vi "产品界面.vi"(8 "错误输入（无错误）":errorcluster, 10 "界面切换队列":refnum<queue>, 11 "VISA资源名称输入":refnum<visa-resource-name>) -> (0 "错误输出":errorcluster, 3 "VISA资源名称输出":refnum<visa-resource-name>)   [LabVIEW 2018]
panel:
  out "毫秒计时值":u32
  in  "枚举":T1(ring)
  in  "选项卡控件":enum32{"选项卡 1", "选项卡 2"}(tab)
  out "写DT200+主料盘参数界面":bool
  out "写DT203":bool
  out "写R176+读R177":bool
  in  "DT422":u16(ring) items=["禁用值", "无名称1", "无名称2", "无名称3", "无名称4", "无名称5", "无名称6", "无名称7", "无名称8", "无名称9", "无名称10", "无名称11", "无名称12", "无名称13", "无名称14", "无名称15", "无名称16", "无名称17", "无名称18", "无名称19", "无名称20", "无名称21", "无名称22", "无名称23", "无名称24", "无名称25", "无名称26", "无名称27", "无名称28", "无名称29", "无名称30", "无名称31", "无名称32", "无名称33", "无名称34", "无名称35", "无名称36", "无名称37", "无名称38", "无名称39", "无名称40", "无名称41", "无名称42", "无名称43", "无名称44", "无名称45", "无名称46", "无名称47", "无名称48", "无名称49", "无名称50", "无名称51", "无名称52", "无名称53", "无名称54", "无名称55", "无名称56", "无名称57", "无名称58", "无名称59", "55UYFJJI"]
  in  "DT420":u16(ring) items=["禁用值", "无名称1", "无名称2", "无名称3", "无名称4", "无名称5", "无名称6", "无名称7", "无名称8", "无名称9", "无名称10", "无名称11", "无名称12", "无名称13", "无名称14", "无名称15", "无名称16", "无名称17", "无名称18", "无名称19", "无名称20", "无名称21", "无名称22", "无名称23", "无名称24", "无名称25", "无名称26", "无名称27", "无名称28", "无名称29", "无名称30", "无名称31", "无名称32", "无名称33", "无名称34", "无名称35", "无名称36", "无名称37", "无名称38", "无名称39", "无名称40", "无名称41", "无名称42", "无名称43", "无名称44", "无名称45", "无名称46", "无名称47", "无名称48", "无名称49", "无名称50", "无名称51", "无名称52", "无名称53", "无名称54", "无名称55", "无名称56", "无名称57", "无名称58", "无名称59", "55UYFJJI"]
  out "字符串 2":string
  in  "产品名称":u16(ring) items=["禁用值", "无名称1", "无名称2", "无名称3", "无名称4", "无名称5", "无名称6", "无名称7", "无名称8", "无名称9", "无名称10", "无名称11", "无名称12", "无名称13", "无名称14", "无名称15", "无名称16", "无名称17", "无名称18", "无名称19", "无名称20", "无名称21", "无名称22", "无名称23", "无名称24", "无名称25", "无名称26", "无名称27", "无名称28", "无名称29", "无名称30", "无名称31", "无名称32", "无名称33", "无名称34", "无名称35", "无名称36", "无名称37", "无名称38", "无名称39", "无名称40", "无名称41", "无名称42", "无名称43", "无名称44", "无名称45", "无名称46", "无名称47", "无名称48", "无名称49", "无名称50", "无名称51", "无名称52", "无名称53", "无名称54", "无名称55", "无名称56", "无名称57", "无名称58", "无名称59", "55UYFJJI"]
  out "DDT90356":dbl
  out "DDT90348":dbl
  out "自动界面":bool
  out "手动界面":bool
  out "参数界面":bool
  out "IO界面":bool
  out "产品界面":bool
  out "字符串":string
  out "DDT90352":dbl
  out "DDT90360":dbl
  out "DT1184":T2(ring)
  out "通讯周期":dbl
  out "数值":dbl
  # "X"
  # "Z1"
  # "XXXXX自动化设备有限公司"
  # "Z2"
  # "Y"
  # "调用"
  # "设置"
  # "编号"
  # "名称"
  # "将产品"
  # "复制到"
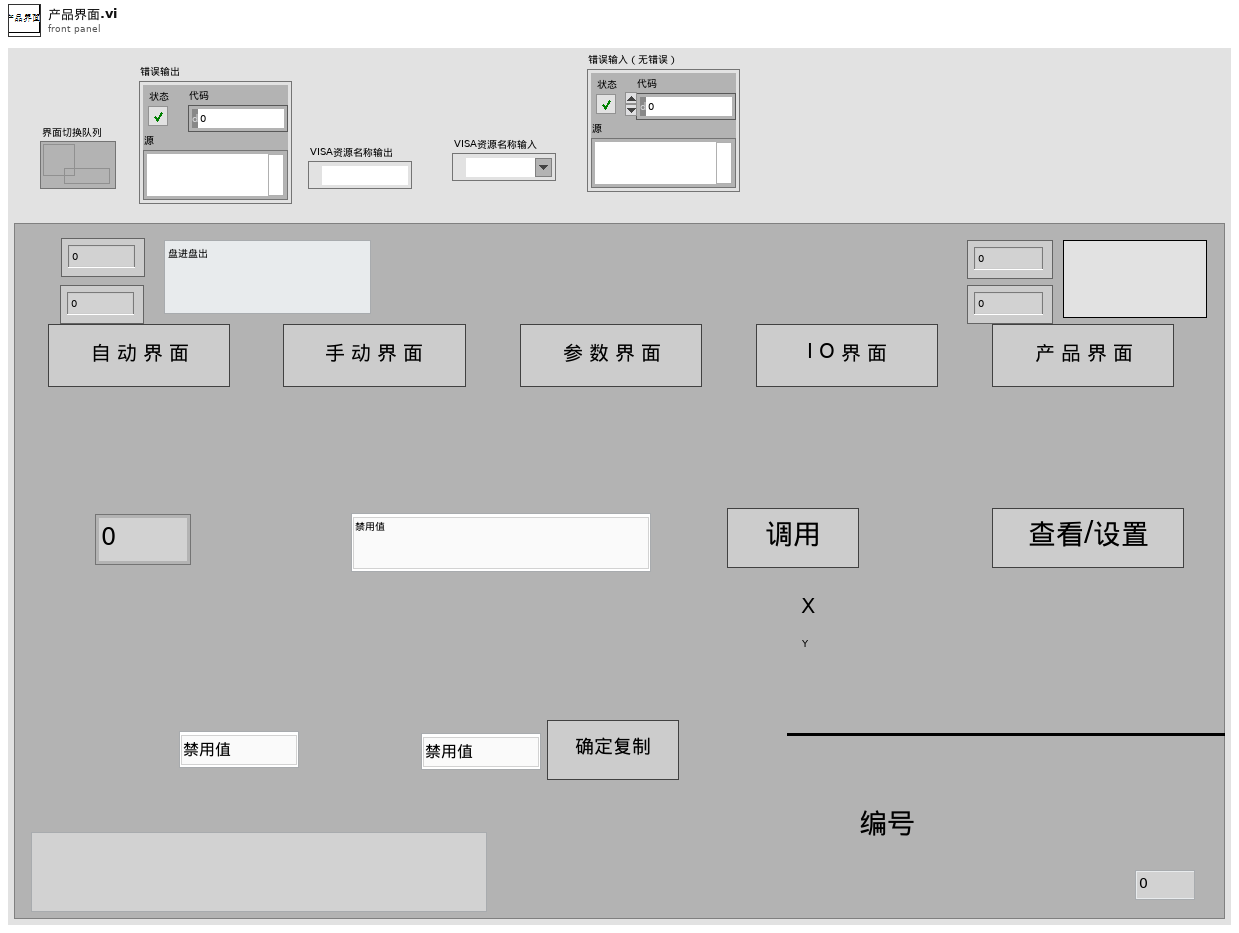
[diagram p1: front panel]
types:
  T1 = enum16{"读初始化", "读R166+8", "读DT420+10", "读R177+8", "读DDT90356", "读DT1184", "读DDT90348", ""}
  T2 = enum16{"盘进盘出", "卷进卷出", "盘进卷出", "管进盘出", "管进卷出", "卷进盘出", ""}
  T3 = enum8{"Enabled", "Disabled", "Disabled and Grayed Out"}
  T4 = typedef "数据簇.ctl" = cluster{"字符串":string, "数值":i32, "布尔":bool}
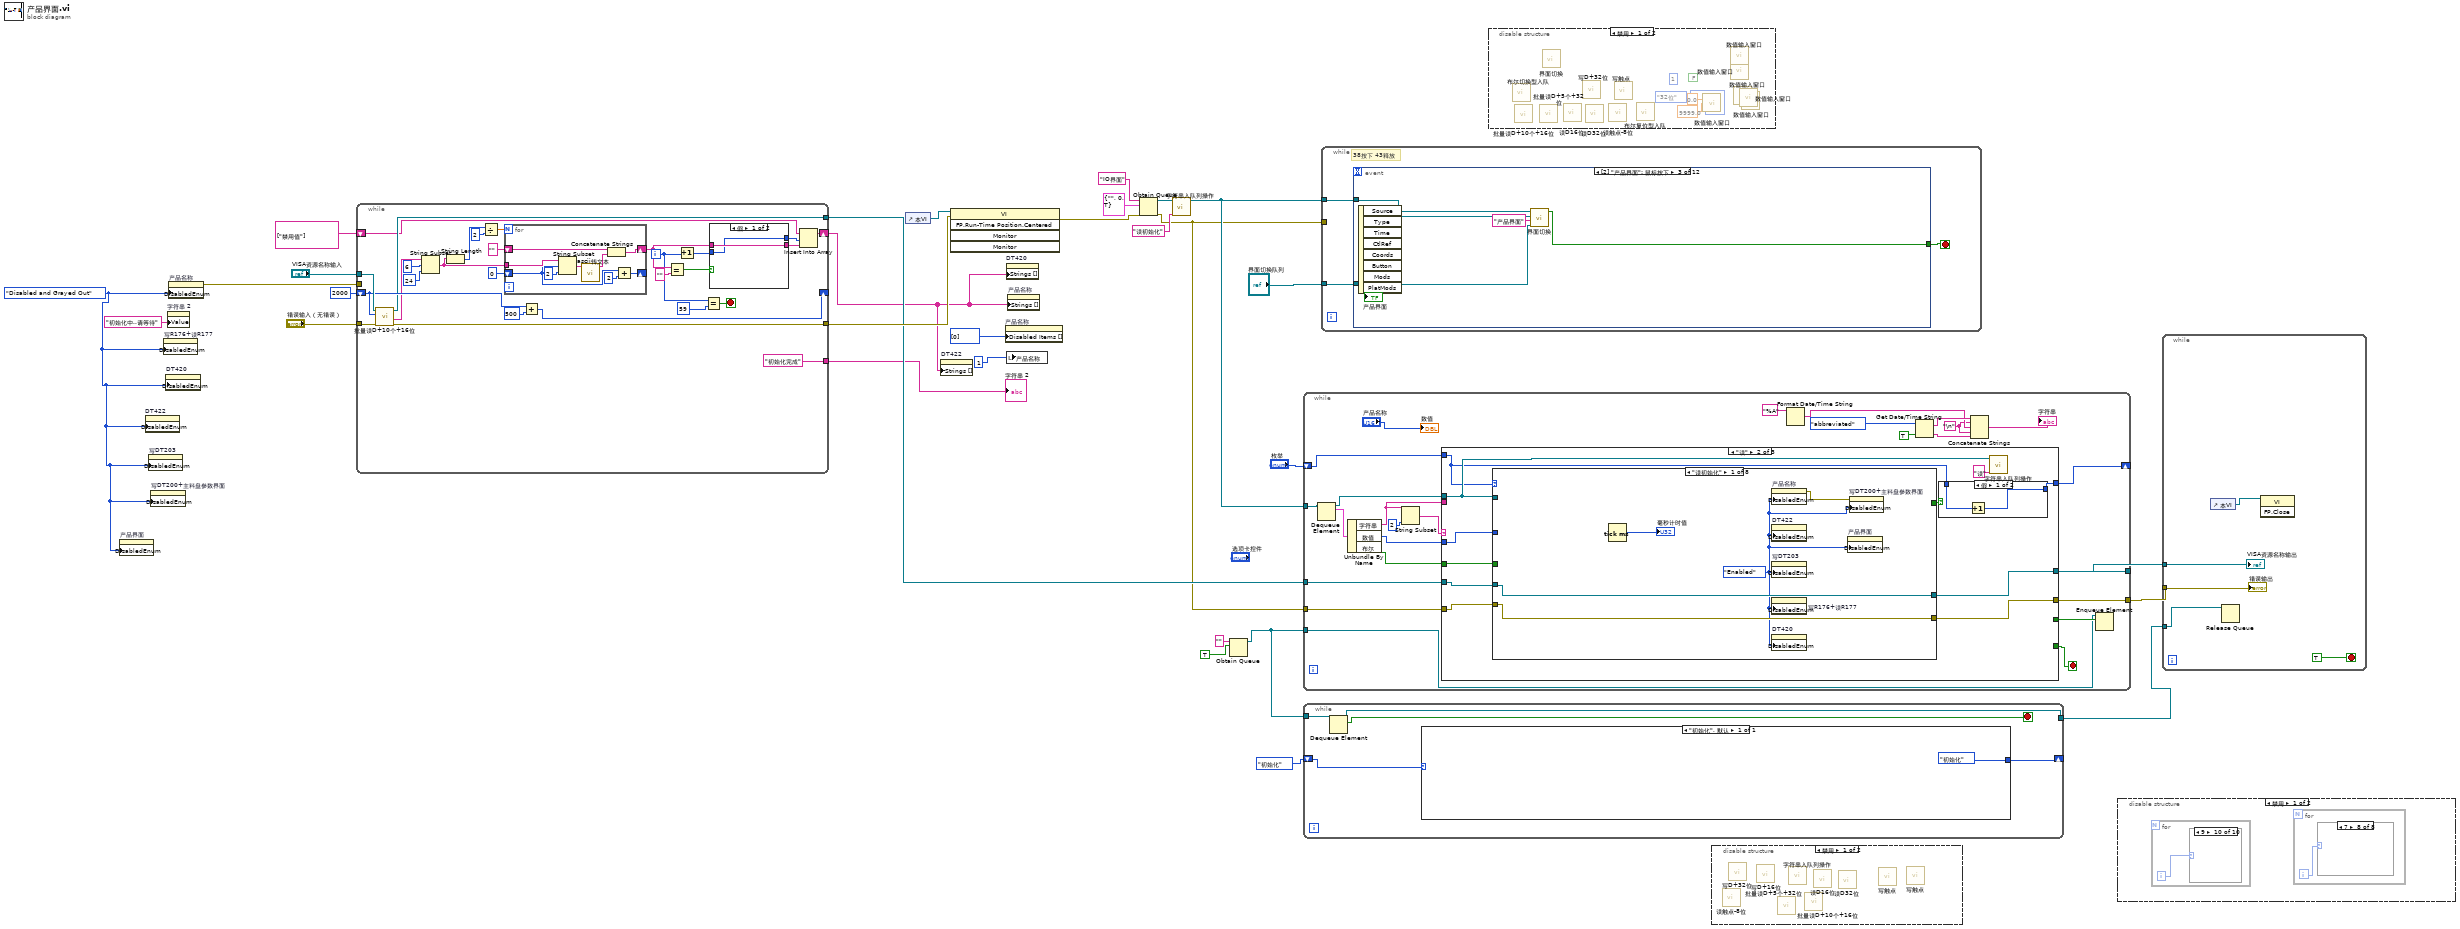
[diagram p0: block diagram]
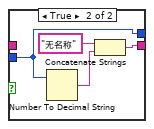
[diagram p2: hidden frame]
diagram:
  w1 = T3."Disabled and Grayed Out" ("禁用")
  n1 = property on="产品界面" class="Bool"("DisabledEnum"=w1) -> ()  [unwired: 2 in, 2 out]
  n2 = property on="DT422" class="Ring (严格)"("DisabledEnum"=w1) -> ()  [unwired: 2 in, 2 out]
  n3 = property on="写DT203" class="Bool"("DisabledEnum"=w1) -> ()  [unwired: 2 in, 2 out]
  n4 = property on="写DT200+主料盘参数界面" class="Bool"("DisabledEnum"=w1) -> ()  [unwired: 2 in, 2 out]
  n5 = property on="写R176+读R177" class="Bool"("DisabledEnum"=w1) -> ()  [unwired: 2 in, 2 out]
  n6 = property on="DT420" class="Ring (严格)"("DisabledEnum"=w1) -> ()  [unwired: 2 in, 2 out]
  n7 = property on="字符串 2" class="Str"("Value"="初始化中..请等待" ("字符串 2")) -> ()  [unwired: 2 in, 2 out]
  n8 = property on="产品名称" class="Ring (严格)"("DisabledEnum"=w1) -> (error out=w2:errorcluster)  [unwired: 2 in, 1 out]
  n9 = while {
    tunnel: "VISA资源名称输入" -> [w58]
    tunnel: "错误输入（无错误）" -> [w57]
    tunnel: [w50] -> w12
    shift-right: [w55] -> _
    shift-left: 2000 -> [w54]
    tunnel: [w51] -> w10
    shift-right: [w39] -> w4
    shift-left: string[] ["禁用值"] -> [w40]
    tunnel: ["初始化完成" ("字符串 2")] -> w6
    tunnel: w2 -> [_]
    i -> [w32]
    stop <- w52 stop-if-true
    n10 = call "批量读D+10个+16位.vi"("error out"=w57, "读取D地址"=w54, "VISA resource name out"=w58) -> ("error IO"=w50:errorcluster, "读取缓冲区"=w41:string, "VISA resource name out 2"=w51:refnum<visa-resource-name>)  [unwired: 5 in, 1 out]
    n11 = String Subset(string=w41, offset (0)=6 ("偏移量(0)"), length (rest)=24 ("长度（剩余）")) -> (substring=w49:string)
    n12 = String Length(string=w49) -> (length=w47:i32)
    n13 = Divide(x=w47, y=2) -> (x/y=w48:dbl)
    n14 = for {
      N: w48 -> [_]
      shift-right: [w65] -> w36
      shift-left: "" -> [w67]
      tunnel: w49 -> [w73]
      shift-right: [w69] -> _
      shift-left: 0 -> [w68]
      n15 = String Subset(string=w73, offset (0)=w68, length (rest)=2 ("长度（剩余）")) -> (substring=w72:string)
      n16 = call "ascii转文本.vi"("输入"=w72) -> ("输出"=w66:string)  [unwired: 9 in, 1 out]
      n17 = Concatenate Strings(w67, w66) -> (w65:string)
      n18 = Add(x=w68, y=2) -> (x+y=w69:i32)
    }
    n19 = Add(x=w54, y=500) -> (x+y=w55:i32)
    n20 = Equal?(x=w36, y="") -> (x = y?=w37:bool)
    n21 = Increment(x=w32) -> (x+1=w33:i32)
    n22 = Equal?(x=w32, y=59) -> (x = y?=w52:bool)
    n23 = case shown="假" w37 {
      tunnel: [w60 w61] -> w35
      tunnel: w36 -> [w60 _]
      tunnel: w33 -> [w59 w64]
      tunnel: [w59 w64] -> w34
      frame False {
      }
      frame True {
        n24 = Number To Decimal String(number=w64) -> (decimal integer string=w62:string)  [unwired: 1 in]
        n25 = Concatenate Strings("无名称" ("字符串"), w62) -> (w61:string)
      }
    }
    n26 = Insert Into Array(array=w40, index=w34, new element=w35) -> (w39:string[])
  }
  "字符串 2" <- w6
  n27 = control-ref of="本VI"() -> (w16:refnum<vi>)
  n28 = property on="DT422" class="Ring (严格)"("Strings []"=w4) -> ()  [unwired: 2 in, 2 out]
  n29 = invoke class="VI" method="FP.Run-Time Position.Centered"(reference=w16, error in=w12) -> (error out=w15:errorcluster)  [unwired: 3 in, 4 out]
  n30 = property on="产品名称" class="Ring (严格)"("Disabled Items []"=i32[] [0] ("禁用项[]")) -> ()  [unwired: 2 in, 2 out]
  n31 = property on="DT420" class="Ring (严格)"("Strings []"=w4) -> ()  [unwired: 2 in, 2 out]
  n32 = local write "产品名称"(1) -> ()
  n33 = property on="产品名称" class="Ring (严格)"("Strings []"=w4) -> ()  [unwired: 2 in, 2 out]
  n34 = Obtain Queue(name (unnamed)="IO界面" ("名称（未命名）"), element data type=T4 {"字符串"="", "数值"=0, "布尔"=TRUE}, error in (no error)=w15) -> (queue out=w25:refnum<queue>, error out=w9:errorcluster)  [unwired: 2 in, 1 out]
  n35 = call "字符串入队列操作.vi"("字符消息入队列"="读初始化", "界面切换队列"=w25) -> ("队列输出"=w17:refnum<queue>)  [unwired: 9 in]
  n36 = Obtain Queue(name (unnamed)="" ("名称（未命名）"), element data type=TRUE) -> (queue out=w20:refnum<queue>)  [unwired: 3 in, 2 out]
  n37 = while {
    tunnel: w17 -> [w95]
    tunnel: w10 -> [w88]
    tunnel: w9 -> [w87]
    tunnel: [w86] -> w27
    tunnel: [w85] -> w26
    shift-right: [w82] -> _
    shift-left: "枚举" -> [w83]
    tunnel: w20 -> [w75]
    stop <- w77 stop-if-true
    w79 = "\n"
    n38 = Dequeue Element(queue=w95) -> (queue out=w92:refnum<queue>, element=w94:T4)  [unwired: 2 in, 2 out]
    n39 = Unbundle By Name(w94) -> ("字符串"=w89:string, "数值"=w91:i32, "布尔"=w90:bool)
    n40 = String Subset(string=w89, length (rest)=2 ("长度（剩余）")) -> (substring=w93:string)  [unwired: 1 in]
    n41 = case shown="\"读\"" w93 {
      selector: w93 -> [w102 _ _]
      tunnel: w92 -> [_ w110 w214]
      tunnel: w91 -> [_ w117 w213]
      tunnel: w90 -> [_ w116 w212]
      tunnel: w89 -> [_ _ w206]
      tunnel: w88 -> [w101 w115 w211]
      tunnel: w87 -> [w100 w114 w210]
      tunnel: [w101 w113 w208] -> w86
      tunnel: [w100 w112 w207] -> w85
      tunnel: [_ _ w209] -> w77
      tunnel: w83 -> [_ w108 _]
      tunnel: [_ w107 _] -> w82
      tunnel: [_ _ w204] -> w76
      frame "", Default {
        n42 = Concatenate Strings("无对应消息分支**" ("消息"), w102, "**" ("字符串"), "读写状态机" ("字符串")) -> (w104:string)
        n43 = One Button Dialog(message=w104) -> ()  [unwired: 1 in, 1 out]
      }
      frame "读" {
        n44 = case shown="\"读初始化\"" w108 {
          tunnel: w110 -> [_ _ _ _ _ _ _ _]
          tunnel: w117 -> [_ _ _ _ _ _ _ _]
          tunnel: w115 -> [w124 w130 w141 w156 w165 w178 w190 w197]
          tunnel: w114 -> [w123 w129 w140 w155 w164 w177 w189 w196]
          tunnel: [w124 w128 w137 w154 w163 w176 w190 w193] -> w113
          tunnel: [w123 w127 w136 w153 w162 w175 w189 w192] -> w112
          tunnel: w116 -> [_ _ _ _ _ _ _ _]
          tunnel: [_ _ _ _ _ _ TRUE _] -> w109
          frame "读初始化" {
            w120 = T3."Enabled" ("禁用")
            n45 = Tick Count (ms)() -> (millisecond timer value=→"毫秒计时值":u32)
            n46 = property on="产品名称" class="Ring (严格)"("DisabledEnum"=w120) -> (error out=w121:errorcluster)  [unwired: 2 in, 1 out]
            n47 = property on="DT422" class="Ring (严格)"("DisabledEnum"=w120) -> ()  [unwired: 2 in, 2 out]
            n48 = property on="写DT203" class="Bool"("DisabledEnum"=w120) -> ()  [unwired: 2 in, 2 out]
            n49 = property on="写R176+读R177" class="Bool"("DisabledEnum"=w120) -> ()  [unwired: 2 in, 2 out]
            n50 = property on="DT420" class="Ring (严格)"("DisabledEnum"=w120) -> ()  [unwired: 2 in, 2 out]
            n51 = property on="产品界面" class="Bool"("DisabledEnum"=w120) -> ()  [unwired: 2 in, 2 out]
            n52 = property on="写DT200+主料盘参数界面" class="Bool"(error in=w121, "DisabledEnum"=w120) -> ()  [unwired: 1 in, 2 out]
          }
          frame "读DT420+10" {
            n53 = call "批量读D+10个+16位.vi"("error out"=w129, "读取D地址"=420, "VISA resource name out"=w130) -> ("error IO"=w127:errorcluster, "数组"=w125:i32[], "VISA resource name out 2"=w128:refnum<visa-resource-name>)  [unwired: 5 in, 1 out]
            n54 = for {
              tunnel: w125 -> [w131] mode=indexing
              i -> [w132]
              n55 = case shown="2" w132 {
                tunnel: w131 -> [w133 _ w134 _ _ _ _ _ _ _]
                frame 0, Default {
                  n56 = local write "DT420"(w133) -> ()
                }
                frame 1 {
                }
                frame 2 {
                  n57 = local write "DT422"(w134) -> ()
                }
                frame 3 {
                }
                frame 4 {
                }
                frame 5 {
                }
                frame 6 {
                }
                frame 7 {
                }
                frame 8 {
                }
                frame 9 {
                }
              }
            }
          }
          frame "读R177+8" {
            n58 = call "读触点-8位.vi"("error out"=w140, "触点类型"="R", "读取起始地址"="177", "VISA resource name out"=w141) -> ("error IO"=w136:errorcluster, "读取布尔数组"=w135:bool[], "VISA resource name out 2"=w137:refnum<visa-resource-name>)  [unwired: 4 in, 1 out]
            n59 = for {
              tunnel: w135 -> [w142] mode=indexing
              i -> [w143]
              n60 = case shown="0, 默认" w143 {
                tunnel: w142 -> [w144 _ _ _ _ _ _ _]
                frame 0, Default {
                  "写R176+读R177" <- w144
                }
                frame 1 {
                }
                frame 2 {
                }
                frame 3 {
                }
                frame 4 {
                }
                frame 5 {
                }
                frame 6 {
                }
                frame 7 {
                }
              }
            }
          }
          frame "读DDT90356" {
            n61 = call "批量读D+5个+32位.vi"("error out"=w155, "读取D地址"=90356, "VISA resource name out"=w156) -> ("error IO"=w153:errorcluster, "数组"=w159:i32[], "VISA resource name out 2"=w154:refnum<visa-resource-name>)  [unwired: 5 in, 1 out]
            n62 = Index Array(array=w159, index #1=0 ("索引"), index #2=2 ("索引")) -> (element #1=w152:i32, element #2=w151:i32)
            n63 = To Double Precision Float(number=w152) -> (double precision float=w150:dbl)
            n64 = To Double Precision Float(number=w151) -> (double precision float=w147:dbl)
            n65 = Divide(x=w150, y=100.0) -> (x/y=→"DDT90356":dbl)
            n66 = Divide(x=w147, y=100.0) -> (x/y=→"DDT90360":dbl)
          }
          frame "读DT1184" {
            n67 = call "读D16位.vi"("error out"=w164, "读取D地址"=1184, "VISA resource name out"=w165) -> ("error IO"=w162:errorcluster, "数值"=→"DT1184":u32, "VISA resource name out 2"=w163:refnum<visa-resource-name>)  [unwired: 5 in, 1 out]
          }
          frame "读DDT90348" {
            n68 = call "批量读D+5个+32位.vi"("error out"=w177, "读取D地址"=90348, "VISA resource name out"=w178) -> ("error IO"=w175:errorcluster, "数组"=w182:i32[], "VISA resource name out 2"=w176:refnum<visa-resource-name>)  [unwired: 5 in, 1 out]
            n69 = Index Array(array=w182, index #1=0 ("索引"), index #2=2 ("索引")) -> (element #1=w174:i32, element #2=w173:i32)
            n70 = To Double Precision Float(number=w173) -> (double precision float=w168:dbl)
            n71 = To Double Precision Float(number=w174) -> (double precision float=w172:dbl)
            n72 = Divide(x=w168, y=100.0) -> (x/y=→"DDT90352":dbl)
            n73 = Divide(x=w172, y=100.0) -> (x/y=→"DDT90348":dbl)
          }
          frame "" {
            n74 = local read "毫秒计时值"() -> (w186:u32)
            n75 = Tick Count (ms)() -> (millisecond timer value=w187:u32)
            n76 = Subtract(x=w187, y=w186) -> (x-y=w185:u32)
            n77 = Divide(x=w185, y=u32 1000) -> (x/y=→"通讯周期":dbl)
          }
          frame "读R166+8" {
            n78 = call "读触点-8位.vi"("error out"=w196, "触点类型"="R", "读取起始地址"="166", "VISA resource name out"=w197) -> ("error IO"=w192:errorcluster, "读取布尔数组"=w191:bool[], "VISA resource name out 2"=w193:refnum<visa-resource-name>)  [unwired: 4 in, 1 out]
            n79 = for {
              tunnel: w191 -> [w198] mode=indexing
              i -> [w199]
              n80 = case shown="0, 默认" w199 {
                tunnel: w198 -> [w201 _ _ _ _ _ _ _]
                frame 0, Default {
                  n81 = case shown="假" w201 {
                    tunnel: ["等待调用....." "数据调用中...请等待"] -> w200
                    frame False {
                    }
                    frame True {
                    }
                  }
                  n82 = local write "字符串 2"(w200) -> ()
                }
                frame 1 {
                }
                frame 2 {
                }
                frame 3 {
                }
                frame 4 {
                }
                frame 5 {
                }
                frame 6 {
                }
                frame 7 {
                }
              }
            }
          }
        }
        n83 = case shown="假" w109 {
          tunnel: w108 -> [w119 _]
          tunnel: [w118 _] -> w107
          frame False {
            n84 = Increment(x=w119) -> (x+1=w118:T1)
          }
          frame True {
          }
        }
        n85 = call "字符串入队列操作.vi"("字符消息入队列"="读", "界面切换队列"=w110) -> ()  [unwired: 9 in, 1 out]
      }
      frame "写" {
        n86 = call "状态匹配.vi"("输入状态"=w206) -> ("输出状态"=w205:string)  [unwired: 10 in]
        n87 = case shown="\"写退出\"" w205 {
          selector: w205 -> [w217 _ _ _ _]
          tunnel: w214 -> [_ _ _ _ w257]
          tunnel: w213 -> [_ w223 w240 _ _]
          tunnel: w212 -> [_ _ _ w251 _]
          tunnel: w211 -> [w216 w233 w244 w256 w262]
          tunnel: w210 -> [w215 w232 w243 w255 w261]
          tunnel: [_ _ _ _ w260] -> w209
          tunnel: [w216 w231 w242 w254 w262] -> w208
          tunnel: [w215 w230 w241 w253 w261] -> w207
          tunnel: w206 -> [_ w222 w234 w245 _]
          tunnel: [_ _ _ _ w260] -> w204
          frame "", Default {
            n88 = Concatenate Strings("无对应消息分支**" ("消息"), w217, "**" ("字符串"), "写状态机" ("字符串")) -> (w221:string)
            n89 = One Button Dialog(message=w221) -> ()  [unwired: 1 in, 1 out]
          }
          frame "写DT" {
            n90 = String Length(string=w222) -> (length=w228:i32)
            n91 = Subtract(x=w228, y=4) -> (x-y=w226:i32)
            n92 = String Subset(string=w222, offset (0)=4 ("偏移量(0)"), length (rest)=w226) -> (substring=w225:string)
            n93 = Decimal String To Number(string=w225) -> (number=w224:i32)  [unwired: 2 in, 1 out]
            n94 = call "写D+16位.vi"("error out"=w232, "输入数值"=w223, "输入地址D"=w224, "VISA resource name out"=w233) -> ("error out 2"=w230:errorcluster, "VISA resource name out 2"=w231:refnum<visa-resource-name>)  [unwired: 3 in, 3 out]
          }
          frame "写DDT" {
            n95 = String Length(string=w234) -> (length=w238:i32)
            n96 = Subtract(x=w238, y=5) -> ()  [unwired: 1 out]
            n97 = String Subset(string=w234, offset (0)=5 ("偏移量(0)")) -> (substring=w235:string)  [unwired: 1 in]
            n98 = Decimal String To Number(string=w235) -> (number=w236:i32)  [unwired: 2 in, 1 out]
            n99 = call "写D+32位.vi"("error out"=w243, "输入数值"=w240, "输入地址D"=w236, "VISA resource name out"=w244) -> ("error out 2"=w241:errorcluster, "VISA resource name out 2"=w242:refnum<visa-resource-name>)  [unwired: 4 in, 2 out]
          }
          frame "写R" {
            n100 = String Length(string=w245) -> (length=w249:i32)
            n101 = Subtract(x=w249, y=3) -> (x-y=w247:i32)
            n102 = String Subset(string=w245, offset (0)=3 ("偏移量(0)"), length (rest)=w247) -> (substring=w246:string)
            n103 = call "写触点.vi"("布尔"=w251, "error out"=w255, "触点类型"="R", "写入起始地址"=w246, "VISA resource name out"=w256) -> ("error IO"=w253:errorcluster, "VISA resource name out 2"=w254:refnum<visa-resource-name>)  [unwired: 4 in, 1 out]
          }
          frame "写退出" {
            w260 = TRUE
            n104 = Flush Queue(queue=w257) -> (queue out=w258:refnum<queue>, error out=w259:errorcluster)  [unwired: 1 in, 1 out]
            n105 = Release Queue(queue=w258, error in (no error)=w259) -> ()  [unwired: 1 in, 3 out]
          }
        }
      }
    }
    n106 = Format Date/Time String(time format string (%c)="%A" ("时间格式字符串(%c)")) -> (date/time string=w80:string)  [unwired: 2 in]
    n107 = Get Date/Time String(date format (0)=enum16{"short", "long", "abbreviated"}."abbreviated" ("日期格式(0)"), want seconds? (F)=TRUE ("需要秒？(F)")) -> (date string=w97:string, time string=w78:string)  [unwired: 1 in]
    n108 = Concatenate Strings(w97, w79, w80, w79, w78) -> (→"字符串":string)
    n109 = Enqueue Element(queue=w75, element=w76) -> ()  [unwired: 2 in, 3 out]
    "数值" <- "产品名称"
  }
  n110 = while {
    shift-right: [w266] -> _
    shift-left: enum16{"初始化"}."初始化" -> [w267]
    tunnel: w20 -> [w265]
    tunnel: [w263] -> w19
    stop <- w264 stop-if-true
    n111 = Dequeue Element(queue=w265) -> (queue out=w263:refnum<queue>, element=w264:bool)  [unwired: 2 in, 2 out]
    n112 = case shown="\"初始化\", 默认" w267 {
      tunnel: [enum16{"初始化"}."初始化"] -> w266
      frame "初始化", Default {
      }
    }
  }
  n113 = while {
    tunnel: w17 -> [w270]
    tunnel: "界面切换队列" -> [w269]
    tunnel: w9 -> [_]
    stop <- w271 stop-if-true
    # "38按下 43释放"
    n114 = event shown="[2] \"产品界面\": 鼠标按下" {
      selector: _ -> [_ _ _ _ _ _ _ _ _ _ _ _]
      dyn-events: _ -> [_ _ _ _ _ _ _ _ _ _ _ _]
      timeout: _ -> [_ _ _ _ _ _ _ _ _ _ _ _]
      tunnel: [w275 w277 w282 w288 _ _ _ _ w326 w331 _ w338] -> w271
      tunnel: w270 -> [w276 w281 w286 w295 w300 w303 w306 w317 w330 w335 _ w337]
      tunnel: w269 -> [w274 w280 w285 w290 _ _ _ _ w329 w334 _ w336]
      event "IO界面": Mouse Down {
        n115 = event-data() -> ("CtlRef"=w273:refnum<vi>)  [unwired: 1 in, 7 out]
        n116 = call "界面切换.vi"("界面切换队列输入"=w274, "切换界面名称输入"="IO界面", "Bool引用句柄"=w273, "状态转移输入"=w276) -> ("布尔"=w275:bool)  [unwired: 7 in]
      }
      event "参数界面": Mouse Down {
        n117 = event-data() -> ("CtlRef"=w279:refnum<vi>)  [unwired: 1 in, 7 out]
        n118 = call "界面切换.vi"("界面切换队列输入"=w280, "切换界面名称输入"="参数界面", "Bool引用句柄"=w279, "状态转移输入"=w281) -> ("布尔"=w277:bool)  [unwired: 7 in]
      }
      event "产品界面": Mouse Down {
        n119 = event-data() -> ("CtlRef"=w284:refnum<vi>)  [unwired: 1 in, 7 out]
        n120 = call "界面切换.vi"("界面切换队列输入"=w285, "切换界面名称输入"="产品界面", "Bool引用句柄"=w284, "状态转移输入"=w286) -> ("布尔"=w282:bool)  [unwired: 7 in]
      }
      event "写DT200+主料盘参数界面": Mouse Down {
        n121 = event-data() -> ("CtlRef"=w287:refnum<vi>)  [unwired: 1 in, 7 out]
        n122 = local read "产品名称"() -> (w293:u16)
        n123 = call "字符串入队列操作.vi"("字符消息入队列"="写DT200", "数值"=w293, "界面切换队列"=w295) -> ("队列输出"=w294:refnum<queue>)  [unwired: 8 in]
        n124 = flat-sequence {
          tunnel: w294 -> [w297]
          tunnel: [w297] -> w291
          frame #0 {
            n125 = Wait (ms)(milliseconds to wait=u32 50 ("等待时间（毫秒）")) -> ()  [unwired: 1 out]
          }
        }
        n126 = call "界面切换.vi"("界面切换队列输入"=w290, "切换界面名称输入"="主料盘参数界面", "Bool引用句柄"=w287, "状态转移输入"=w291) -> ("布尔"=w288:bool)  [unwired: 7 in]
      }
      event "DT420": Value Change {
        n127 = event-data() -> ("NewVal"=w298:u16)  [unwired: 1 in, 5 out]
        n128 = call "字符串入队列操作.vi"("字符消息入队列"="写DT420", "数值"=w298, "界面切换队列"=w300) -> ()  [unwired: 8 in, 1 out]
      }
      event "DT422": Value Change {
        n129 = event-data() -> ("NewVal"=w302:u16)  [unwired: 1 in, 5 out]
        n130 = call "字符串入队列操作.vi"("字符消息入队列"="写DT422", "数值"=w302, "界面切换队列"=w303) -> ()  [unwired: 8 in, 1 out]
      }
      event "写DT203": Mouse Down {
        n131 = event-data() -> ()  [unwired: 1 in, 8 out]
        n132 = property on="产品名称" class="Ring (严格)"() -> ("RingText.Text"=w304:string)  [unwired: 2 in, 2 out]
        n133 = Concatenate Strings("确定调用产品" ("消息"), "\n", w304) -> (w308:string)
        n134 = Two Button Dialog(message=w308) -> (T button?=w307:bool)  [unwired: 2 in]
        n135 = case shown="真" w307 {
          tunnel: w306 -> [_ w312]
          frame False {
          }
          frame True {
            n136 = local read "产品名称"() -> (w311:u16)
            n137 = call "字符串入队列操作.vi"("字符消息入队列"="写DT203", "数值"=w311, "界面切换队列"=w312) -> ()  [unwired: 8 in, 1 out]
          }
        }
      }
      event "写R176+读R177": Mouse Down {
        w314 = "\n"
        n138 = event-data() -> ("CtlRef"=w316:refnum<vi>)  [unwired: 1 in, 7 out]
        n139 = property on="DT422" class="Ring (严格)"() -> ("RingText.Text"=w313:string)  [unwired: 2 in, 2 out]
        n140 = property on="DT420" class="Ring (严格)"() -> ("RingText.Text"=w320:string)  [unwired: 2 in, 2 out]
        n141 = Concatenate Strings("确定将" ("字符串"), w314, w320, w314, "复制到" ("字符串"), w314, w313) -> (w319:string)
        n142 = Two Button Dialog(message=w319) -> (T button?=w318:bool)  [unwired: 2 in]
        n143 = case shown="真" w318 {
          tunnel: w317 -> [_ w325]
          tunnel: w316 -> [_ w324]
          frame False {
          }
          frame True {
            n144 = call "布尔切换型入队.vi"("字符串"="写R176", "true启用入队"=TRUE, "控件引用"=w324, "消息入队列"=w325) -> ()  [unwired: 8 in]
          }
        }
      }
      event "手动界面": Mouse Down {
        n145 = event-data() -> ("CtlRef"=w328:refnum<vi>)  [unwired: 1 in, 7 out]
        n146 = call "界面切换.vi"("界面切换队列输入"=w329, "切换界面名称输入"="手动界面", "Bool引用句柄"=w328, "状态转移输入"=w330) -> ("布尔"=w326:bool)  [unwired: 7 in]
      }
      event "自动界面": Mouse Down {
        n147 = event-data() -> ("CtlRef"=w333:refnum<vi>)  [unwired: 1 in, 7 out]
        n148 = call "界面切换.vi"("界面切换队列输入"=w334, "切换界面名称输入"="自动界面", "Bool引用句柄"=w333, "状态转移输入"=w335) -> ("布尔"=w331:bool)  [unwired: 7 in]
      }
      event Timeout {
        n149 = event-data() -> ()  [unwired: 1 in, 3 out]
      }
      event Panel Close? {
        n150 = event-data() -> ()  [unwired: 1 in, 4 out]
        n151 = Two Button Dialog(message="确定退出程序？" ("消息")) -> (T button?=w339:bool)  [unwired: 2 in]
        n152 = case shown="真" w339 {
          tunnel: [_ TRUE] -> w338
          tunnel: w337 -> [_ w344]
          tunnel: w336 -> [_ w343]
          frame False {
          }
          frame True {
            n153 = call "字符串入队列操作.vi"("字符消息入队列"="退出", "界面切换队列"=w343) -> ()  [unwired: 9 in, 1 out]
            n154 = call "字符串入队列操作.vi"("字符消息入队列"="写退出", "界面切换队列"=w344) -> ()  [unwired: 9 in, 1 out]
          }
        }
        n155 = event-data("Discard?"=TRUE ("放弃？")) -> ()  [unwired: 1 in, 1 out]
      }
    }
  }
  n156 = disable-structure shown="禁用" {
    frame Disabled {
      (unwired) u32 1 ("转换比例")
      (unwired) FALSE ("忽略数值上下限")
      n157 = call "布尔切换型入队.vi"() -> ()  [unwired: 12 in]
      n158 = call "批量读D+10个+16位.vi"() -> ()  [unwired: 8 in, 4 out]
      n159 = call "批量读D+5个+32位.vi"() -> ()  [unwired: 8 in, 4 out]
      n160 = call "界面切换.vi"() -> ()  [unwired: 11 in, 1 out]
      n161 = call "读D16位.vi"() -> ()  [unwired: 8 in, 4 out]
      n162 = call "写D+32位.vi"() -> ()  [unwired: 8 in, 4 out]
      n163 = call "读D32位.vi"() -> ()  [unwired: 9 in, 3 out]
      n164 = call "读触点-8位.vi"() -> ()  [unwired: 8 in, 4 out]
      n165 = call "写触点.vi"() -> ()  [unwired: 9 in, 3 out]
      n166 = call "布尔复位型入队.vi"() -> ()  [unwired: 6 in, 3 out]
      n167 = call "数值输入窗口.vi"("输入下限"=0.0, "输入上限"=9999.0, "数据类型"=enum16{"32位", "16位"}."32位") -> ("转换比例"=w350:u32)  [unwired: 9 in, 3 out]
      n168 = call "数值输入窗口.vi"() -> ()  [unwired: 13 in, 3 out]
      n169 = call "数值输入窗口.vi"() -> ()  [unwired: 13 in, 3 out]
      n170 = call "数值输入窗口.vi"() -> ()  [unwired: 13 in, 3 out]
      n171 = call "数值输入窗口.vi"() -> ()  [unwired: 13 in, 3 out]
      n172 = call "数值输入窗口.vi"() -> ()  [unwired: 13 in, 3 out]
    }
    frame Enabled {
    }
  }
  n173 = disable-structure shown="禁用" {
    frame Disabled {
      n174 = call "读触点-8位.vi"() -> ()  [unwired: 8 in, 4 out]
      n175 = call "写D+32位.vi"() -> ()  [unwired: 8 in, 4 out]
      n176 = call "写D+16位.vi"() -> ()  [unwired: 7 in, 5 out]
      n177 = call "批量读D+5个+32位.vi"() -> ()  [unwired: 8 in, 4 out]
      n178 = call "字符串入队列操作.vi"() -> ()  [unwired: 11 in, 1 out]
      n179 = call "批量读D+10个+16位.vi"() -> ()  [unwired: 8 in, 4 out]
      n180 = call "读D16位.vi"() -> ()  [unwired: 8 in, 4 out]
      n181 = call "读D32位.vi"() -> ()  [unwired: 9 in, 3 out]
      n182 = call "写触点.vi"() -> ()  [unwired: 9 in, 3 out]
      n183 = call "写触点.vi"() -> ()  [unwired: 9 in, 3 out]
    }
    frame Enabled {
    }
  }
  n184 = disable-structure shown="禁用" {
    frame Disabled {
      n185 = for {
        i -> [w352]
        n186 = case shown="9" w352 {
          frame 0, Default {
          }
          frame 1 {
          }
          frame 2 {
          }
          frame 3 {
          }
          frame 4 {
          }
          frame 5 {
          }
          frame 6 {
          }
          frame 7 {
          }
          frame 8 {
          }
          frame 9 {
          }
        }
      }
      n187 = for {
        i -> [w351]
        n188 = case shown="7" w351 {
          frame 0, Default {
          }
          frame 1 {
          }
          frame 2 {
          }
          frame 3 {
          }
          frame 4 {
          }
          frame 5 {
          }
          frame 6 {
          }
          frame 7 {
          }
        }
      }
    }
    frame Enabled {
    }
  }
  n189 = while {
    tunnel: w27 -> [w355]
    tunnel: w26 -> [w354]
    tunnel: w19 -> [w353]
    stop <- TRUE stop-if-true
    n190 = control-ref of="本VI"() -> (w356:refnum<vi>)
    n191 = Release Queue(queue=w353) -> ()  [unwired: 2 in, 3 out]
    n192 = invoke class="VI" method="FP.Close"(reference=w356) -> ()  [unwired: 2 in, 3 out]
    "VISA资源名称输出" <- w355
    "错误输出" <- w354
  }
